vi "disdrometer_dataparse.vi"(11 "Poll Response":string) -> (4 "Complete Dataset":string[](array[string]), 8 "output cluster":T1, 10 "Spectrum Data":dbl[](array[numeric]))   [LabVIEW 2018]
doc: "Given a poll response from the Thies Clima disdrometer, deciphers the response string into arrays. Available ouputs include the complete dataset array, or subarrays seperated into general data, spectrum data, and debug data."
uses:
  Epimedia_Connex_Source/HDF5/DisdromterSummaryData.ctl
panel:
  out "ToDisplay":dbl[](array[numeric])
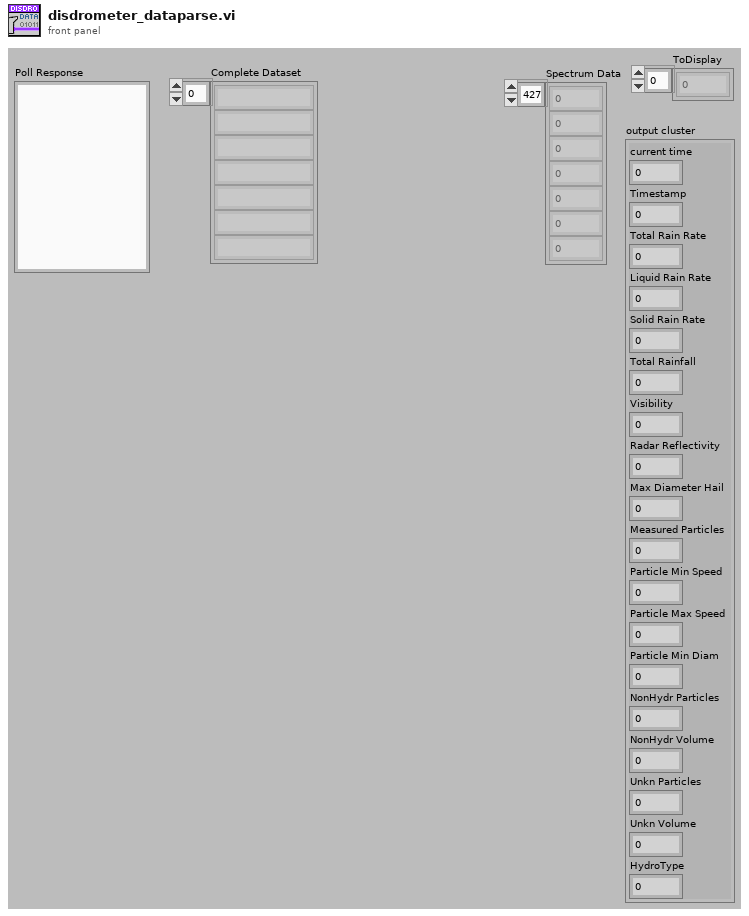
[diagram p1: front panel]
types:
  T1 = typedef "DisdromterSummaryData.ctl" = cluster{"current time":dbl, "Timestamp":dbl, "Total Rain Rate":dbl, "Liquid Rain Rate":dbl, "Solid Rain Rate":dbl, "Total Rainfall":dbl, "Visibility":dbl, "Radar Reflectivity":dbl, "Max Diameter Hail":dbl, "Measured Particles":i16, "Particle Min Speed":i16, "Particle Max Speed":i16, "Particle Min Diam":i16, "NonHydr Particles":i16, "NonHydr Volume":dbl, "Unkn Particles":i16, "Unkn Volume":dbl, "HydroType":i8}
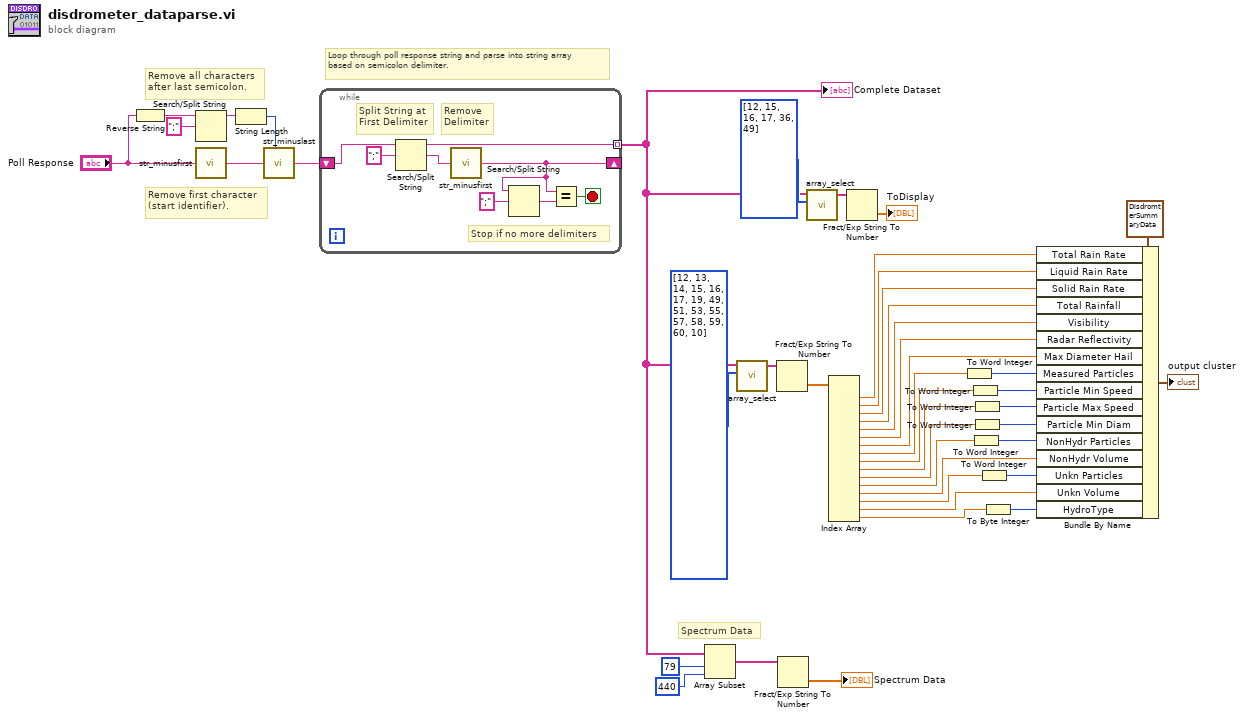
[diagram p0: block diagram]
diagram:
  # "Spectrum Data"
  # "Remove all characters\nafter last semicolon."
  # "Remove first character\n(start identifier)."
  # "Loop through poll response string and parse into string array\nbased on semicolon delimiter."
  n1 = Reverse String(1:"Poll Response") -> (0:w39:string)
  n2 = Search/Split String(string=w39, search string/char (-)=";") -> (substring before match=w38:string)  [unwired: 1 in, 2 out]
  n3 = call "str_minusfirst.vi"("String In"="Poll Response") -> ("String Out"=w43:string)  [unwired: 6 in]
  n4 = String Length(string=w38) -> (length=w37:i32)
  n5 = call "str_minuslast.vi"("N"=w37, "String In"=w43) -> ("String Out"=w42:string)  [unwired: 5 in]
  n6 = while {
    tunnel: [w50] -> w28 mode=indexing
    shift-right: [w44] -> _
    shift-left: w42 -> [w49]
    stop <- w48 stop-if-true
    # "Stop if no more delimiters"
    # "Remove\nDelimiter"
    # "Split String at\nFirst Delimiter"
    n7 = Search/Split String(string=w49, search string/char (-)=";") -> (substring before match=w50:string, match + rest of string=w47:string)  [unwired: 1 in, 1 out]
    n8 = call "str_minusfirst.vi"("String In"=w47) -> ("String Out"=w44:string)  [unwired: 6 in]
    n9 = Search/Split String(string=w44, search string/char (-)=";") -> (match + rest of string=w46:string)  [unwired: 1 in, 2 out]
    n10 = Equal?(x=w44, y=w46) -> (x = y?=w48:bool)
  }
  "Complete Dataset" <- w28
  n11 = Array Subset(array=w28, index=79, length=440) -> (w16:string[])
  n12 = call "array_select.vi"("Selection"=i32[] [12, 13, 14, 15, 16, 17, 19, 49, 51, 53, 55, 57, 58, 59, 60, 10], "Array In"=w28) -> ("Array Out"=w34:string[])  [unwired: 9 in]
  n13 = Fract/Exp String To Number(string=w34) -> (number=w29:dbl[])  [unwired: 3 in, 1 out]
  n14 = Fract/Exp String To Number(string=w16) -> (number=→"Spectrum Data":dbl[])  [unwired: 3 in, 1 out]
  n15 = call "array_select.vi"("Selection"=i32[] [12, 15, 16, 17, 36, 49], "Array In"=w28) -> ("Array Out"=w31:string[])  [unwired: 9 in]
  n16 = Index Array(array=w29) -> (element #1=w27:dbl, element #2=w26:dbl, element #3=w25:dbl, element #4=w24:dbl, element #5=w23:dbl, element #6=w22:dbl, element #7=w21:dbl, element #8=w20:dbl, element #9=w12:dbl, element #10=w11:dbl, element #11=w10:dbl, element #12=w9:dbl, element #13=w19:dbl, element #14=w3:dbl, element #15=w18:dbl, element #16=w4:dbl)  [unwired: 16 in]
  n17 = Fract/Exp String To Number(string=w31) -> (number=→"ToDisplay":dbl[])  [unwired: 3 in, 1 out]
  n18 = To Word Integer(number=w20) -> (16bit integer=w13:i16)
  n19 = To Word Integer(number=w12) -> (16bit integer=w5:i16)
  n20 = To Word Integer(number=w9) -> (16bit integer=w8:i16)
  n21 = To Word Integer(number=w11) -> (16bit integer=w6:i16)
  n22 = To Word Integer(number=w10) -> (16bit integer=w7:i16)
  n23 = To Word Integer(number=w3) -> (16bit integer=w2:i16)
  n24 = To Byte Integer(number=w4) -> (8bit integer=w1:i8)
  n25 = Bundle By Name(cluster=T1 {"current time"=0.0, "Timestamp"=0.0, "Total Rain Rate"=0.0, "Liquid Rain Rate"=0.0, "Solid Rain Rate"=0.0, "Total Rainfall"=0.0, "Visibility"=0.0, "Radar Reflectivity"=0.0, "Max Diameter Hail"=0.0, "Measured Particles"=0, "Particle Min Speed"=0, "Particle Max Speed"=0, "Particle Min Diam"=0, "NonHydr Particles"=0, "NonHydr Volume"=0.0, "Unkn Particles"=0, "Unkn Volume"=0.0, "HydroType"=0} ("DisdromSummary"), "Total Rain Rate"=w27, "Liquid Rain Rate"=w26, "Solid Rain Rate"=w25, "Total Rainfall"=w24, "Visibility"=w23, "Radar Reflectivity"=w22, "Max Diameter Hail"=w21, "Measured Particles"=w13, "Particle Min Speed"=w5, "Particle Max Speed"=w6, "Particle Min Diam"=w7, "NonHydr Particles"=w8, "NonHydr Volume"=w19, "Unkn Particles"=w2, "Unkn Volume"=w18, "HydroType"=w1) -> (→"output cluster":T1)
